vi "FPGA TEST.vi"() -> ()   [LabVIEW 2023]
uses:
  <vilib>/rvi/Emulation/niFpgaGetClockAttributes.vi
  <vilib>/rvi/Emulation/niFpgaSctlEmulationGetInTimedLoop.vi
  <vilib>/rvi/Emulation/niFpgaEmulationReportErrorSimple.vi
  <vilib>/rvi/eio/common/nirviEmuTemplateMethod_errors.vi
  <vilib>/rvi/Emulation/niFpgaCriticalErrorInLSC.vi
  <vilib>/rvi/Emulation/niFpgaProcessEmulError.vi
  <vilib>/eio/EIONode/EIONode.xnode
panel:
  out "Digital 2":bool=TRUE
  out "Digital 1":bool=TRUE
  in  "Digital 2 ON/OFF":bool
  in  "Digital 1 ON/OFF":bool
  in  "stop 3":bool
  in  "Data":sgl
  in  "State Analog":u8
  in  "stop 2":bool
  out "Running?":bool
  out "Low Time":sgl
  out "High Time":sgl
  in  "State PWM":i32=2
  in  "Duty Cycle\n0-100":sgl
  out "Output 0":bool
  in  "stop":bool
  # "Analog"
  # "PWM"
  # "Digital"
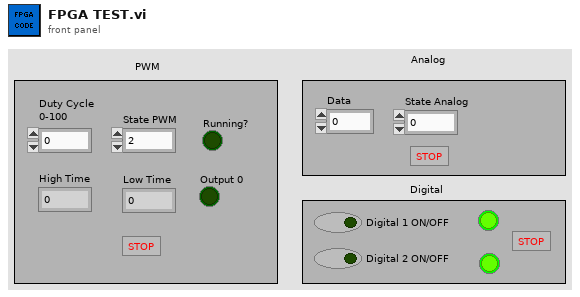
[diagram p1: front panel]
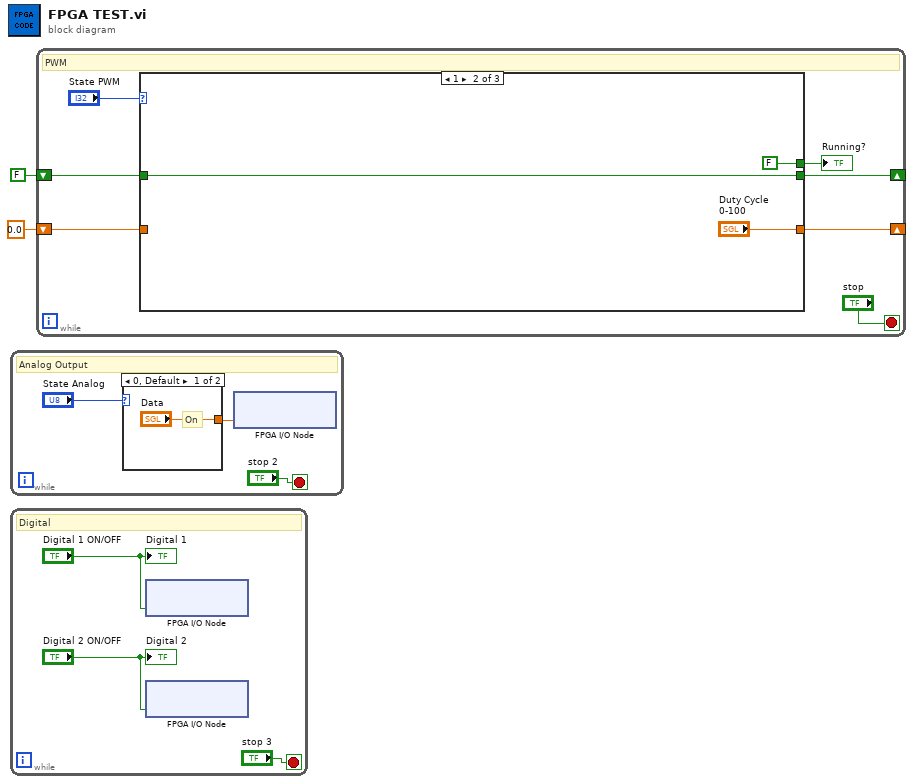
[diagram p0: block diagram]
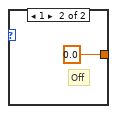
[diagram p2: hidden frame]
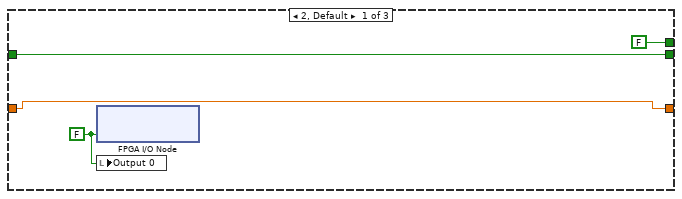
[diagram p3: hidden frame]
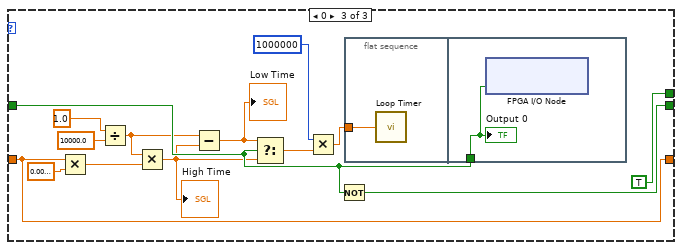
[diagram p4: hidden frame]
diagram:
  n1 = while {
    stop <- "stop 2" stop-if-true
    # "Analog Output"
    n2 = case shown="0, Default" "State Analog" {
      tunnel: ["Data" sgl 0.0 ("Data 2")] -> w3
      frame 0, Default {
        # "On"
      }
      frame 1 {
        # "Off"
      }
    }
    n3 = xnode "FPGA I/O Node"("Mod2/AO0"=w3) -> ()  [unwired: 1 in, 1 out]
  }
  n4 = while {
    stop <- "stop 3" stop-if-true
    # "Digital"
    n5 = xnode "FPGA I/O Node"("Mod1/DO2"="Digital 1 ON/OFF") -> ()  [unwired: 1 in, 1 out]
    n6 = xnode "FPGA I/O Node"("Mod1/DO1"="Digital 2 ON/OFF") -> ()  [unwired: 1 in, 1 out]
    "Digital 1" <- "Digital 1 ON/OFF"
    "Digital 2" <- "Digital 2 ON/OFF"
  }
  n7 = while "PWM Generation" {
    shift-right: [w16] -> _
    shift-left: FALSE -> [w17]
    shift-right: [w13] -> _
    shift-left: sgl 0.0 ("Duty Cycle\n0-100") -> [w14]
    stop <- "stop" stop-if-true
    # "PWM"
    n8 = case shown="1" "State PWM" {
      tunnel: w17 -> [w21 w23 w38]
      tunnel: [w21 w23 w37] -> w16
      tunnel: w14 -> [w20 _ w28]
      tunnel: [w20 "Duty Cycle\n0-100" w28] -> w13
      tunnel: [FALSE FALSE TRUE] -> w11
      frame 2, Default {
        w19 = FALSE ("Mod1/DO0")
        n9 = xnode "FPGA I/O Node"("Mod1/DO0"=w19) -> ()  [unwired: 1 in, 1 out]
        n10 = local write "Output 0"(w19) -> ()
      }
      frame 1 {
      }
      frame 0 {
        n11 = Multiply(x=w28, y=sgl 0.01) -> (x*y=w34:sgl)
        n12 = Divide(x=sgl 1.0, y=sgl 10000.0 ("Frequency (Hz) 2")) -> (x/y=w33:sgl)
        n13 = Multiply(x=w33, y=w34) -> (x*y=w27:sgl)
        "High Time" <- w27
        n14 = Subtract(x=w33, y=w27) -> (x-y=w26:sgl)
        "Low Time" <- w26
        n15 = Select(t=w26, s=w38, f=w27) -> (s? t:f=w32:sgl)
        n16 = Multiply(x=u32 1000000, y=w32) -> (x*y=w30:sgl)
        n17 = Not(x=w38) -> (.not. x?=w37:bool)
        n18 = flat-sequence {
          tunnel: w30 -> [w39]
          tunnel: w38 -> [w40]
          frame #0 {
            n19 = call "Loop Timer"("Count(uSec)"=w39) -> ()  [unwired: 1 out]
          }
          frame #1 {
            n20 = xnode "FPGA I/O Node"("Mod1/DO0"=w40) -> ()  [unwired: 1 in, 1 out]
            "Output 0" <- w40
          }
        }
      }
    }
    "Running?" <- w11
  }
